vi "SaveTracking.vi"(1 "Input Data xyzt":T1, 2 "file_name":string caption="Name :", 3 "file path (dialog if empty)":path) -> ()   [LabVIEW 2018]
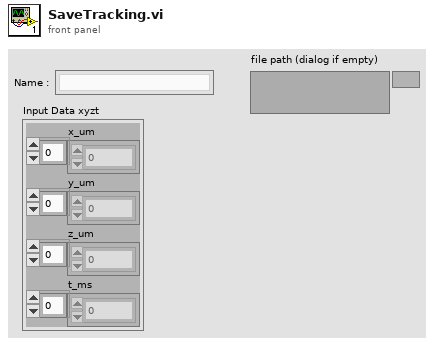
[diagram p1: front panel]
types:
  T1 = cluster{"x_um":sgl[], "y_um":sgl[], "z_um":sgl[], "t_ms":u32[]}
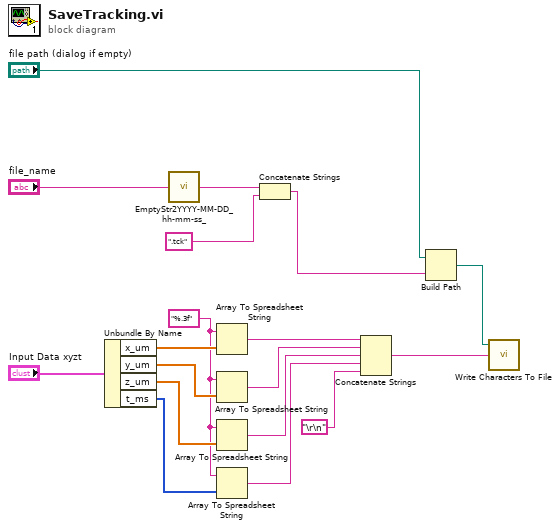
[diagram p0: block diagram]
diagram:
  w12 = "%.3f" ("format string")
  n1 = Unbundle By Name("Input Data xyzt") -> ("x_um"=w16:sgl[], "y_um"=w13:sgl[], "z_um"=w14:sgl[], "t_ms"=w15:u32[])
  n2 = call "EmptyStr2YYYY-MM-DD_hh-mm-ss_.vi"("file_name"="file_name") -> ("OutputName"=w5:string)
  n3 = Array To Spreadsheet String(array=w16, 3:w12) -> (spreadsheet string=w10:string)  [unwired: 1 in]
  n4 = Array To Spreadsheet String(array=w13, 3:w12) -> (spreadsheet string=w9:string)  [unwired: 1 in]
  n5 = Array To Spreadsheet String(array=w14, 3:w12) -> (spreadsheet string=w8:string)  [unwired: 1 in]
  n6 = Array To Spreadsheet String(array=w15, 3:w12) -> (spreadsheet string=w11:string)  [unwired: 1 in]
  n7 = Concatenate Strings(w5, ".tck") -> (w2:string)
  n8 = Concatenate Strings(w10, w9, w8, w11, "\r\n") -> (w18:string)
  n9 = Build Path(base path="file path (dialog if empty)", name or relative path=w2) -> (appended path=w1:path)
  n10 = call <vilib>:"Write Characters To File.vi"("character string"=w18, "file path (dialog if empty)"=w1) -> ()  [unwired: 3 in, 1 out]
